vi "Teleop.vi"(10 "Match Info":T2={"Autonomous Elapsed Seconds"=0.0, "TeleOp Elapsed Seconds"=0.0, "Disabled Elapsed Seconds"=0.0, "Visited Autonomous"=FALSE, "Visited TeleOp"=FALSE, "Visited Disabled"=FALSE, "Autonomous Settings"={"Autonomous Style"=enum."Independent", "VI Refnum"=refnum}}, 11 "Call Context":T3) -> ()   [LabVIEW 2017]
doc: "This VI is called for each enabled TeleOp packet received from the DS. It is typically used to read from joysticks and other inputs and update I/O or setpoints for timed control loops. It should complete and return within 20 milliseconds or risk missing DS packets."
uses:
  <vilib>/Rock Robotics/WPI/DriverStation/WPI_DriverStationDerivedRobotMode.ctl
  <vilib>/Rock Robotics/WPI/DriverStation/WPI_DriverStationMatch Info.ctl
  Support Code/Example Block Data.ctl
  <vilib>/Rock Robotics/WPI/Utilities/WPI_GetSetVariantRefNum.vi
  <vilib>/Rock Robotics/Network Tables/NT Write Boolean Array.vi
  <vilib>/Rock Robotics/Network Tables/NT Write Numeric Array.vi
  <vilib>/Rock Robotics/Network Tables/NT Read Raw.vi
  <vilib>/Rock Robotics/WPI/ThirdParty/Phoenix-LabVIEW/Motor Controller/Get/CTRE_Phoenix_MotorController_GetSelectedSensorData.vi
panel:
  out "value":T1
  out "Block Data":string
  out "Blocks":string
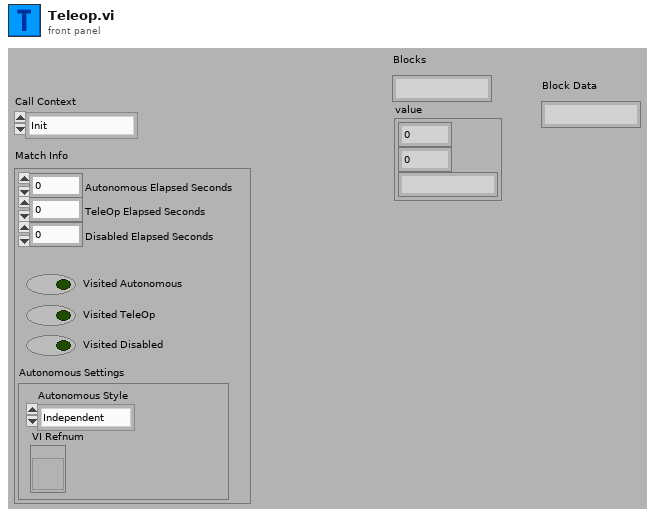
[diagram p1: front panel]
types:
  T1 = typedef "Example Block Data.ctl" = cluster{"Speed":dbl, "Angle":dbl, "Name":string}
  T2 = typedef "WPI_DriverStationMatch Info.ctl" = cluster{"Autonomous Elapsed Seconds":dbl, "TeleOp Elapsed Seconds":dbl, "Disabled Elapsed Seconds":dbl, "Visited Autonomous":bool, "Visited TeleOp":bool, "Visited Disabled":bool, "Autonomous Settings":cluster{"Autonomous Style":enum16{"Iterative", "Independent"}, "VI Refnum":refnum<vi>}}
  T3 = typedef "WPI_DriverStationDerivedRobotMode.ctl" = enum16{"Init", "Execute", "Stop"}
  T4 = typedef "WPI_MotorControlDeviceRef.ctl" = cluster{"DeviceStatus":errorcluster, "Type":T5, "PWM":cluster{"PWM Channel":T6, "DeadBand":T7}, "CAN":cluster{"Device Number":u8, "SetOutput VI Ref":variant, "GetOutput VI Ref":variant, "Enable VI Ref":variant, "Disable VI Ref":variant, "Data":variant}, "Invert":bool, "DIO PWM":cluster{"PWM \"Enable\" Channel":T6, "DIOChannel":T8, "PWM Rate":dbl}}
  T5 = typedef "WPI_MotorControlType.ctl" = enum16{"PWM", "CAN", "DIO PWM"}
  T6 = typedef "FPGA_DIOPWMChannel.ctl" = enum8{"PWM 0", "PWM 1", "PWM 2", "PWM 3", "PWM 4", "PWM 5", "PWM 6", "PWM 7", "PWM 8", "PWM 9", "PWM MXP 0", "PWM MXP 1", "PWM MXP 2", "PWM MXP 3", "PWM MXP 4", "PWM MXP 5", "PWM MXP 6", "PWM MXP 7", "PWM MXP 8", "PWM MXP 9", "Invalid"}
  T7 = typedef "WPI_PWMDeadband.ctl" = cluster{"Name":string, "maxPositivePwm":i32, "minPositivePwm":i32, "centerPwm":i32, "maxNegativePwm":i32, "minNegativePwm":i32, "angularRange":u16}
  T8 = typedef "FPGA_DIOChannel.ctl" = enum8{"DIO 0", "DIO 1", "DIO 2", "DIO 3", "DIO 4", "DIO 5", "DIO 6", "DIO 7", "DIO 8", "DIO 9", "DIO MXP 0", "DIO MXP 1", "DIO MXP 2", "DIO MXP 3", "DIO MXP 4", "DIO MXP 5", "DIO MXP 6", "DIO MXP 7", "DIO MXP 8", "DIO MXP 9", "DIO MXP 10", "DIO MXP 11", "DIO MXP 12", "DIO MXP 13", "DIO MXP 14", "DIO MXP 15", "SPI Port CS1", "SPI Port CS2", "SPI Port CS3", "SPI Port MISO", "SPI Port MOSI", "Invalid"}
  T9 = typedef "WPI_JoystickDevRef.ctl" = cluster{"Device":T10}
  T10 = typedef "WPI_JoystickDeviceEnum.ctl" = enum16{"USB 0", "USB 1", "USB 2", "USB 3", "USB 4", "USB 5"}
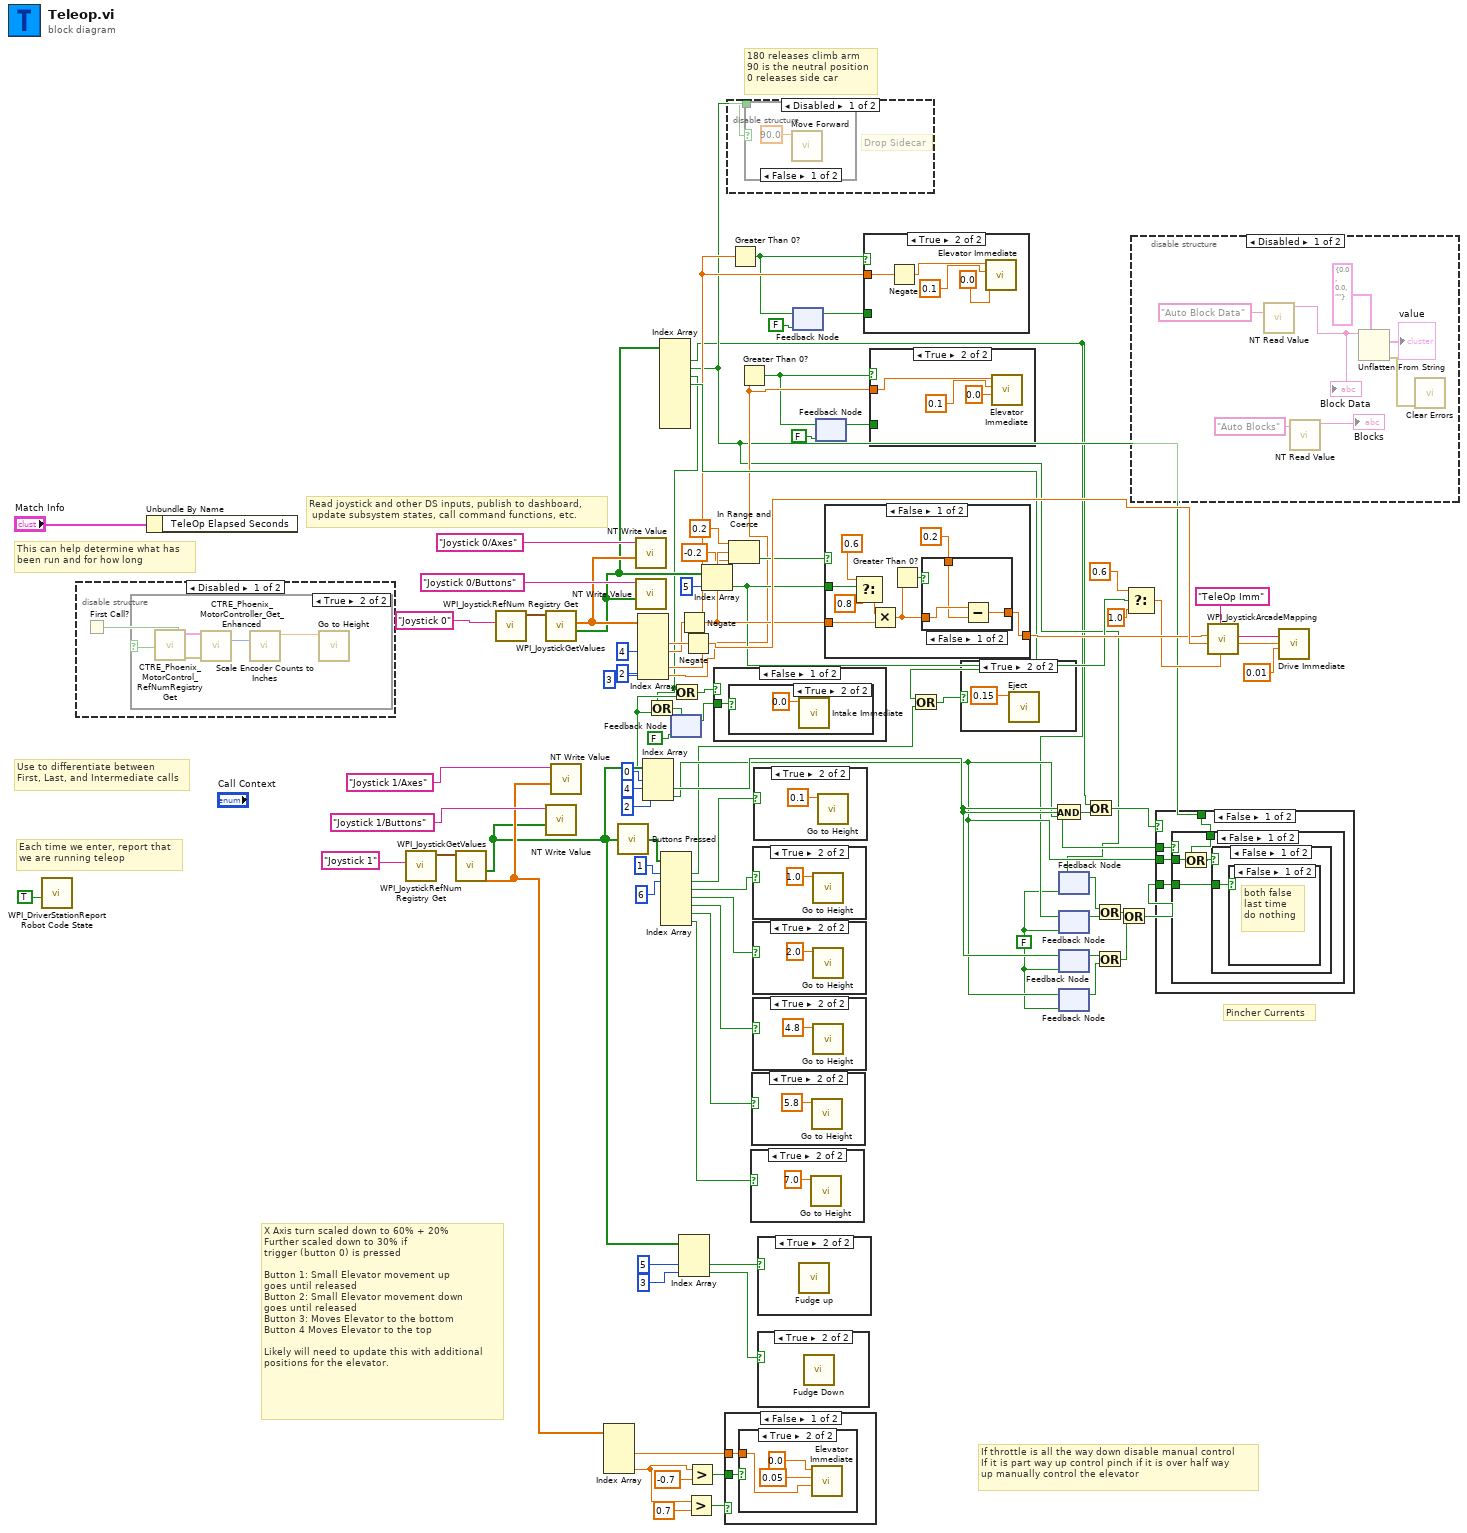
[diagram p0: block diagram]
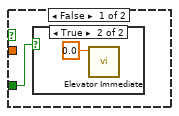
[diagram p2: hidden frame]
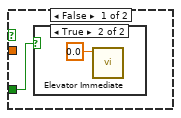
[diagram p4: hidden frame]
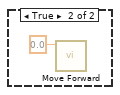
[diagram p6: hidden frame]
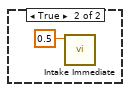
[diagram p12: hidden frame]
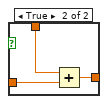
[diagram p13: hidden frame]
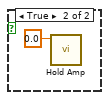
[diagram p16: hidden frame]
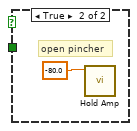
[diagram p17: hidden frame]
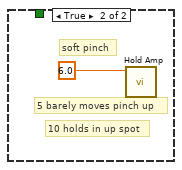
[diagram p18: hidden frame]
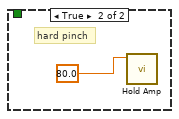
[diagram p19: hidden frame]
diagram:
  w5 = FALSE
  # "180 releases climb arm\n90 is the neutral position\n0 releases side car"
  # "Pincher Currents"
  # "If throttle is all the way down disable manual control\nIf it is part way up control pinch if it is over half way\nup manually control the elevator"
  # "X Axis turn scaled down to 60% + 20%\nFurther scaled down to 30% if\ntrigger (button 0) is pressed\n\nButton 1: Small Elevator movement up\ngoes until released\nButton 2: Small Elevator movement down\ngoes until released\nButton 3: Moves Elevator to the bottom\nButton 4 Moves Elevator to the top\n\nLikely will need to update this with additional\npositions for the elevator."
  # "Read joystick and other DS inputs, publish to dashboard,\n update subsystem states, call command functions, etc."
  # "Each time we enter, report that\nwe are running teleop"
  # "Use to differentiate between\nFirst, Last, and Intermediate calls"
  # "This can help determine what has\nbeen run and for how long"
  n1 = call <vilib>:"WPI_DriverStationReport Robot Code State.vi"("TeleOp"=TRUE ("Autonomous")) -> ()  [unwired: 10 in, 1 out]
  n2 = disable-structure shown="Disabled" {
    frame Disabled {
      n3 = First Call?() -> (First Call?: T/F=w88:bool)
      n4 = case shown="True" w88 {
        frame False {
        }
        frame True {
          n5 = call <vilib>:"CTRE_Phoenix_MotorControl_RefNumRegistryGet.vi"() -> ("error out"=w89:errorcluster, "PhoenixMotorControlDevRef"=w91:T4)  [unwired: 10 in]
          n6 = call-poly <vilib>:"CTRE_Phoenix_MotorController_Get_Enhanced.vi"("PhoenixMotorControlDevRef"=w91, "error in"=w89) -> ("Position (Raw Sensor Units)"=w92:i32)  [unwired: 10 in, 3 out]
          n7 = call "Scale Encoder Counts to Inches.vi"("Target Height (in)"=w92) -> ("Encoder Counts"=w90:dbl)  [unwired: 10 in]
          n8 = call "Go to Height.vi"("Target Height (in)"=w90) -> ()  [unwired: 10 in, 1 out]
        }
      }
    }
    frame Enabled {
    }
  }
  n9 = Unbundle By Name("Match Info") -> ()  [unwired: 1 out]
  n10 = call <vilib>:"WPI_JoystickRefNum Registry Get.vi"("refnum name"="Joystick 1") -> ("JoystickDevRef"=w64:T9)  [unwired: 1 in, 9 out]
  n11 = call <vilib>:"WPI_JoystickGetValues.vi"("JoystickDevRef"=w64) -> ("Buttons"=w42:bool[], "Axes"=w56:dbl[])  [unwired: 6 in, 3 out]
  n12 = call <vilib>:"WPI_JoystickRefNum Registry Get.vi"("refnum name"="Joystick 0") -> ("JoystickDevRef"=w84:T9)  [unwired: 1 in, 9 out]
  n13 = call <vilib>:"WPI_JoystickGetValues.vi"("JoystickDevRef"=w84) -> ("Buttons"=w33:bool[], "Axes"=w82:dbl[])  [unwired: 6 in, 3 out]
  n14 = call-poly <vilib>:"NT Write Value.vi"("Boolean Array"=w42, "Name"="Joystick 1/Buttons") -> ()  [unwired: 9 in, 1 out]
  n15 = call-poly <vilib>:"NT Write Value.vi"("Numeric Array"=w56, "Name"="Joystick 1/Axes") -> ()  [unwired: 9 in, 1 out]
  n16 = Index Array(array=w56) -> (element #2=w55:dbl, element #4=w50:dbl)  [unwired: 4 in, 2 out]
  n17 = call "Buttons Pressed.vi"("Button Values"=w42) -> ("Button Presses"=w77:bool[])
  n18 = call-poly <vilib>:"NT Write Value.vi"("Numeric Array"=w82, "Name"="Joystick 0/Axes") -> ()  [unwired: 9 in, 1 out]
  n19 = call-poly <vilib>:"NT Write Value.vi"("Boolean Array"=w33, "Name"="Joystick 0/Buttons") -> ()  [unwired: 9 in, 1 out]
  n20 = Index Array(array=w82, index #3=4 ("index"), index #5=2 ("index"), index #6=3 ("index")) -> (element #2=w80:dbl, element #3=w78:dbl, element #5=w17:dbl, element #6=w16:dbl)  [unwired: 3 in, 2 out]
  n21 = Index Array(array=w42, index #1=0 ("index"), index #2=4 ("index"), index #3=2 ("index")) -> (element #1=w24:bool, element #2=w40:bool, element #3=w39:bool)
  n22 = Index Array(array=w33) -> (element #1=w6:bool, element #2=w7:bool, element #3=w8:bool, element #4=w20:bool)  [unwired: 9 in, 5 out]
  n23 = Or(x=w8, y=w24) -> (x .or. y?=w9:bool)
  n24 = Index Array(array=w77, index #1=1 ("index"), index #2=6 ("index")) -> (element #1=w21:bool, element #2=w76:bool, element #3=w75:bool, element #4=w49:bool, element #5=w48:bool, element #6=w47:bool, element #7=w46:bool)  [unwired: 5 in]
  n25 = feedback-in #1(w9) -> ()
  n26 = feedback #1(FALSE) -> (w34:bool)
  n27 = Or(x=w8, y=w24) -> (x .or. y?=w23:bool)
  n28 = Negate(x=w78) -> (-x=w59:dbl)
  n29 = Index Array(array=w42, index #2=5 ("index"), index #3=3 ("index")) -> (element #2=w74:bool, element #3=w73:bool)  [unwired: 1 in, 1 out]
  n30 = Negate(x=w80) -> (-x=w79:dbl)
  n31 = Greater?(x=w50, y=0.7) -> (0:w53:bool)
  n32 = Greater?(x=w50, y=-0.7) -> (0:w51:bool)
  n33 = Index Array(array=w33, index=5) -> (element=w31:bool)
  n34 = case shown="False" w23 {
    tunnel: w34 -> [w93 _]
    frame False {
      n35 = case shown="True" w93 {
        frame False {
        }
        frame True {
          n36 = call "Intake Immediate.vi"("Setpoint"=0.0) -> ()  [unwired: 10 in, 1 out]
        }
      }
    }
    frame True {
      n37 = call "Intake Immediate.vi"("Setpoint"=0.5) -> ()  [unwired: 10 in, 1 out]
    }
  }
  n38 = case shown="False" w53 {
    tunnel: w55 -> [w96 w105]
    tunnel: w51 -> [w97 _]
    frame False {
      n39 = case shown="True" w97 {
        tunnel: w96 -> [_ w98]
        frame False {
        }
        frame True {
          n40 = call "Elevator Immediate.vi"("Setpoint Pinch"=w98, "Deadband Value"=0.05, "Setpoint"=0.0 ("Setpoint Pinch")) -> ()  [unwired: 8 in, 1 out]
        }
      }
    }
    frame True {
      n41 = Multiply(x=0.6 ("y"), y=w105) -> (x*y=w102:dbl)
      n42 = call "Elevator Immediate.vi"("Setpoint Pinch"=0.0, "Deadband Value"=0.15, "Setpoint"=w102) -> ()  [unwired: 8 in, 1 out]
    }
  }
  n43 = disable-structure shown="Disabled" {
    disable-tunnel: w7 -> [w106 _]
    frame Disabled {
      # "Drop Sidecar"
      n44 = case shown="False" w106 {
        frame False {
          n45 = call "Move Forward.vi"("Setpoint"=90.0) -> ()  [unwired: 10 in, 1 out]
        }
        frame True {
          n46 = call "Move Forward.vi"("Setpoint"=0.0) -> ()  [unwired: 10 in, 1 out]
        }
      }
    }
    frame Enabled {
    }
  }
  n47 = In Range and Coerce(upper limit=0.2, x=w59, lower limit=-0.2) -> (In Range?=w60:bool)  [unwired: 1 out]
  n48 = Greater Than 0?(x=w17) -> (x > 0?=w10:bool)
  n49 = Greater Than 0?(x=w16) -> (x > 0?=w11:bool)
  n50 = case shown="True" w46 {
    frame False {
    }
    frame True {
      n51 = call "Go to Height.vi"("Target Height (in)"=7.0 ("Setpoint")) -> ()  [unwired: 10 in, 1 out]
    }
  }
  n52 = case shown="True" w47 {
    frame False {
    }
    frame True {
      n53 = call "Go to Height.vi"("Target Height (in)"=5.8 ("Setpoint")) -> ()  [unwired: 10 in, 1 out]
    }
  }
  n54 = case shown="True" w75 {
    frame False {
    }
    frame True {
      n55 = call "Go to Height.vi"("Target Height (in)"=1.0 ("Setpoint")) -> ()  [unwired: 10 in, 1 out]
    }
  }
  n56 = case shown="True" w49 {
    frame False {
    }
    frame True {
      n57 = call "Go to Height.vi"("Target Height (in)"=2.0 ("Setpoint")) -> ()  [unwired: 10 in, 1 out]
    }
  }
  n58 = case shown="True" w48 {
    frame False {
    }
    frame True {
      n59 = call "Go to Height.vi"("Target Height (in)"=4.8 ("Setpoint")) -> ()  [unwired: 10 in, 1 out]
    }
  }
  n60 = case shown="True" w76 {
    frame False {
    }
    frame True {
      n61 = call "Go to Height.vi"("Target Height (in)"=0.1 ("Setpoint")) -> ()  [unwired: 10 in, 1 out]
    }
  }
  n62 = case shown="True" w74 {
    frame False {
    }
    frame True {
      n63 = call "Fudge up.vi"() -> ()  [unwired: 11 in, 1 out]
    }
  }
  n64 = case shown="True" w73 {
    frame False {
    }
    frame True {
      n65 = call "Fudge Down.vi"() -> ()  [unwired: 11 in, 1 out]
    }
  }
  n66 = feedback #2(FALSE) -> (w13:bool)
  n67 = feedback-in #2(w10) -> ()
  n68 = feedback #3(FALSE) -> (w12:bool)
  n69 = feedback-in #3(w11) -> ()
  n70 = case shown="False" w60 {
    tunnel: w59 -> [w123 w130]
    tunnel: w31 -> [w122 _]
    tunnel: [w116 w130] -> w71
    frame False {
      n71 = Select(t=0.6, s=w122, f=0.8) -> (s? t:f=w119:dbl)
      n72 = Multiply(x=w119, y=w123) -> (x*y=w118:dbl)
      n73 = Greater Than 0?(x=w118) -> (x > 0?=w117:bool)
      n74 = case shown="False" w117 {
        tunnel: w118 -> [w125 w129]
        tunnel: [w126 w128] -> w116
        tunnel: 0.2 ("x") -> [w124 w127]
        frame False {
          n75 = Subtract(x=w125, y=w124) -> (x-y=w126:dbl)
        }
        frame True {
          n76 = Add(x=w127, y=w129) -> (x+y=w128:dbl)
        }
      }
    }
    frame True {
    }
  }
  n77 = case shown="True" w10 {
    tunnel: w17 -> [_ w136]
    tunnel: w13 -> [w131 _]
    frame False {
      n78 = case shown="True" w131 {
        frame False {
        }
        frame True {
          n79 = call "Elevator Immediate.vi"("Setpoint"=0.0) -> ()  [unwired: 10 in, 1 out]
        }
      }
    }
    frame True {
      n80 = Negate(x=w136) -> (-x=w135:dbl)
      n81 = call "Elevator Immediate.vi"("Setpoint Pinch"=0.0, "Deadband Value"=0.1, "Setpoint"=w135) -> ()  [unwired: 8 in, 1 out]
    }
  }
  n82 = case shown="True" w11 {
    tunnel: w16 -> [_ w141]
    tunnel: w12 -> [w137 _]
    frame False {
      n83 = case shown="True" w137 {
        frame False {
        }
        frame True {
          n84 = call "Elevator Immediate.vi"("Setpoint"=0.0) -> ()  [unwired: 10 in, 1 out]
        }
      }
    }
    frame True {
      n85 = call "Elevator Immediate.vi"("Setpoint Pinch"=0.0, "Deadband Value"=0.1, "Setpoint"=w141) -> ()  [unwired: 8 in, 1 out]
    }
  }
  n86 = Or(x=w20, y=w21) -> (x .or. y?=w22:bool)
  n87 = case shown="True" w22 {
    frame False {
    }
    frame True {
      n88 = call "Eject.vi"("Setpoint"=0.15 ("Eject Power")) -> ()  [unwired: 10 in, 1 out]
    }
  }
  n89 = And(x=w40, y=w39) -> (x .and. y?=w27:bool)
  n90 = feedback #4(w5) -> (w4:bool)
  n91 = feedback-in #4(w7) -> ()
  n92 = feedback #5(w5) -> (w3:bool)
  n93 = feedback-in #5(w6) -> ()
  n94 = feedback #6(w5) -> (w43:bool)
  n95 = feedback-in #6(w40) -> ()
  n96 = feedback-in #7(w39) -> ()
  n97 = feedback #7(w5) -> (w44:bool)
  n98 = Or(x=w6, y=w27) -> (x .or. y?=w26:bool)
  n99 = Or(x=w4, y=w3) -> (x .or. y?=w1:bool)
  n100 = Or(x=w43, y=w44) -> (x .or. y?=w45:bool)
  n101 = Or(x=w1, y=w45) -> (x .or. y?=w2:bool)
  n102 = Select(t=0.6, s=w31, f=1.0) -> (s? t:f=w28:dbl)
  n103 = disable-structure shown="Disabled" {
    frame Disabled {
      n104 = call-poly <vilib>:"NT Read Value.vi"("Name"="Auto Block Data") -> ("Raw"=w146:string)  [unwired: 9 in, 1 out]
      "Block Data" <- w146
      n105 = call-poly <vilib>:"NT Read Value.vi"("Name"="Auto Blocks") -> ("Raw"=→"Blocks":string)  [unwired: 9 in, 1 out]
      n106 = Unflatten From String(type=T1 {"Speed"=0.0, "Angle"=0.0, "Name"=""} ("Test Cluster"), binary string=w146) -> (value=→"value":T1, error out=w143:errorcluster)  [unwired: 3 in, 1 out]
      n107 = call <vilib>:"Clear Errors.vi"("error in (no error)"=w143) -> ()  [unwired: 5 in, 2 out]
    }
    frame Enabled {
    }
  }
  n108 = case shown="False" w26 {
    tunnel: w40 -> [w153 _]
    tunnel: w39 -> [w152 _]
    tunnel: w2 -> [w151 _]
    tunnel: w7 -> [w150 _]
    frame False {
      n109 = case shown="False" w153 {
        tunnel: w152 -> [w155 _]
        tunnel: w151 -> [w157 _]
        tunnel: w150 -> [w154 _]
        frame False {
          n110 = Or(x=w154, y=w155) -> (x .or. y?=w156:bool)
          n111 = case shown="False" w156 {
            tunnel: w157 -> [w158 _]
            frame False {
              n112 = case shown="False" w158 {
                frame False {
                  # "both false\nlast time\ndo nothing"
                }
                frame True {
                  n113 = call "Hold Amp.vi"("Setpoint"=0.0) -> ()  [unwired: 10 in, 1 out]
                }
              }
            }
            frame True {
              # "open pincher"
              n114 = call "Hold Amp.vi"("Setpoint"=-80.0 ("5")) -> ()  [unwired: 10 in, 1 out]
            }
          }
        }
        frame True {
          # "10 holds in up spot"
          # "5 barely moves pinch up"
          # "soft pinch"
          n115 = call "Hold Amp.vi"("Setpoint"=6.0 ("4")) -> ()  [unwired: 10 in, 1 out]
        }
      }
    }
    frame True {
      # "hard pinch"
      n116 = call "Hold Amp.vi"("Setpoint"=80.0 ("Both")) -> ()  [unwired: 10 in, 1 out]
    }
  }
  n117 = call <vilib>:"WPI_JoystickArcadeMapping.vi"("Max Output"=w28, "Y axis value"=w79, "X axis value"=w71) -> ("Right Motor Value"=w68:dbl, "Left Motor Value"=w69:dbl)  [unwired: 7 in]
  n118 = call "Drive Immediate.vi"("Description"="TeleOp Imm", "Deadband Value"=0.01, "Right Setpoint"=w68, "Left Setpoint"=w69) -> ()  [unwired: 7 in, 1 out]
